vi "Visualize.vi"(8 "error in":errorcluster, 11 "Fast Tree in":refnum<class "Fast Tree.lvclass">) -> (0 "error out":errorcluster, 2 "Visualized Tree":string, 3 "Fast Tree out":refnum<class "Fast Tree.lvclass">)   [LabVIEW 2019, in "Fast Tree.lvclass"]
uses:
  Fast Tree.lvclass
  Fast Tree.lvclass/Fast Tree.ctl
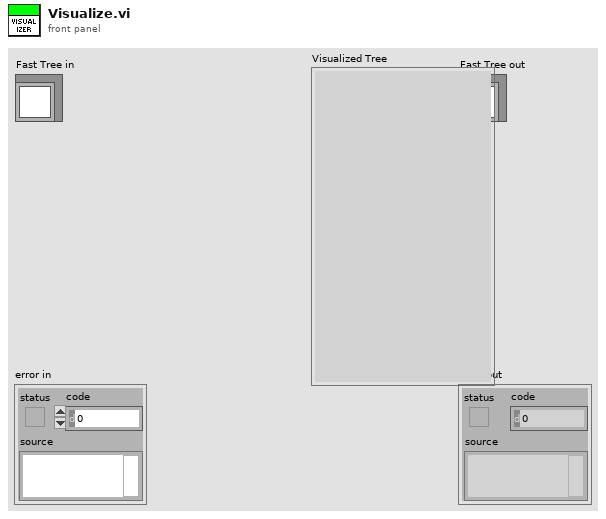
[diagram p1: front panel]
types:
  T1 = cluster{"Record Type":string, "Payload":string, "Parent Index":i32, "First Child Index":i32, "Next Sibling Index":i32}[]
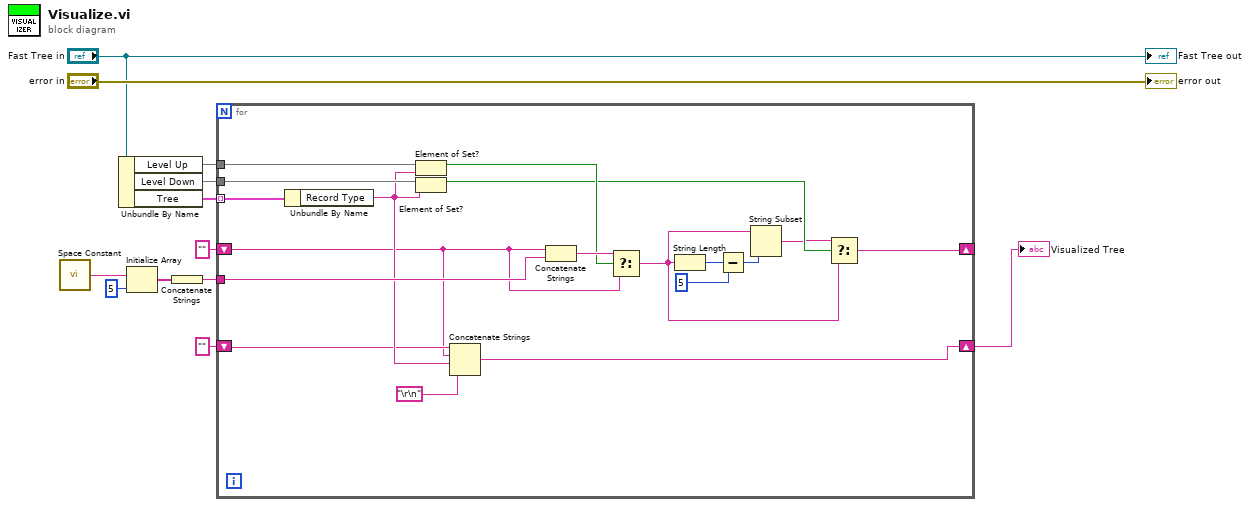
[diagram p0: block diagram]
diagram:
  n1 = call <vilib>:"Space Constant.vi"() -> ("String"=w9:string)
  n2 = Unbundle By Name("Fast Tree in") -> ("Level Up"=w3:set{string}, "Level Down"=w4:set{string}, "Tree"=w10:T1)
  n3 = Initialize Array(w9, 5 ("dimension size")) -> (w7:string[])
  n4 = Concatenate Strings(w7) -> (w6:string)
  n5 = for {
    tunnel: w10 -> [w30] mode=indexing
    tunnel: w6 -> [w28]
    tunnel: w4 -> [w29]
    shift-right: [w20] -> _
    shift-left: "" -> [w19]
    tunnel: w3 -> [w27]
    shift-right: [w25] -> w1
    shift-left: "" -> [w24]
    n6 = Unbundle By Name(w30) -> ("Record Type"=w26:string)
    n7 = Element of Set?(10:w26, 11:w27) -> (3:w17:bool)
    n8 = Element of Set?(10:w26, 11:w29) -> (3:w16:bool)
    n9 = Concatenate Strings(w24, w19, w26, "\r\n") -> (w25:string)
    n10 = Concatenate Strings(w19, w28) -> (w18:string)
    n11 = Select(t=w18, s=w17, f=w19) -> (s? t:f=w13:string)
    n12 = String Length(string=w13) -> (length=w22:i32)
    n13 = Subtract(x=w22, y=5) -> (x-y=w15:i32)
    n14 = String Subset(string=w13, length (rest)=w15) -> (substring=w14:string)  [unwired: 1 in]
    n15 = Select(t=w14, s=w16, f=w13) -> (s? t:f=w20:string)
  }
  "Visualized Tree" <- w1
  "error out" <- "error in"
  "Fast Tree out" <- "Fast Tree in"
